vi "Get File Infor.vi"(8 "error in (no error)":errorcluster, 11 "File Operate Interface in":refnum<class "File Operate Interface.lvclass">) -> (0 "error out":errorcluster, 3 "File Operate Interface out":refnum<class "File Operate Interface.lvclass">)   [LabVIEW 2020, in "File Operate Interface.lvclass"]
uses:
  File Operate Interface.lvclass
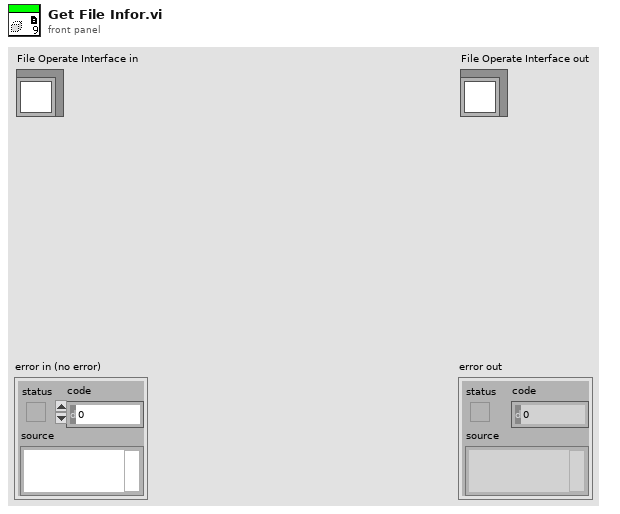
[diagram p1: front panel]
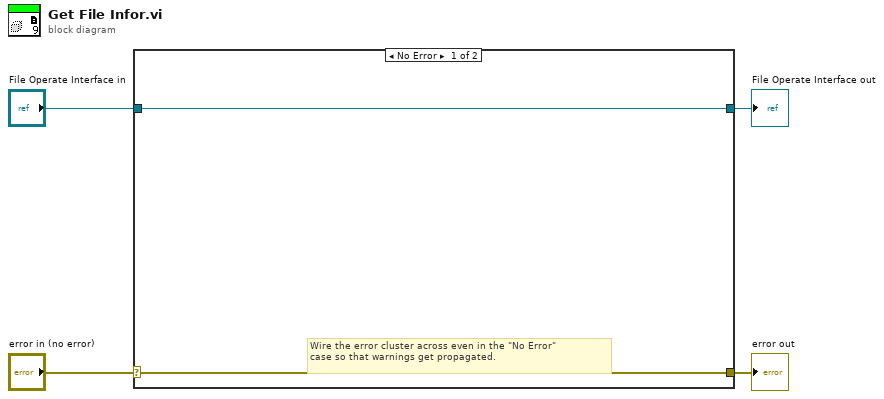
[diagram p0: block diagram]
diagram:
  n1 = case shown="No Error" "error in (no error)" {
    selector: "error in (no error)" -> [w5 w8]
    tunnel: [w5 w8] -> w3
    tunnel: [w6 w7] -> w1
    tunnel: "File Operate Interface in" -> [w6 w7]
    frame No Error {
      # "Wire the error cluster across even in the \"No Error\"\ncase so that warnings get propagated."
    }
    frame Error {
    }
  }
  "error out" <- w3
  "File Operate Interface out" <- w1
